vi "is_bool.vi"(11 "data in":string) -> (1 "confirmed?":bool, 3 "data out":variant)   [LabVIEW 2020, in "configuration-data.lvclass"]
uses:
  configuration-data.lvclass
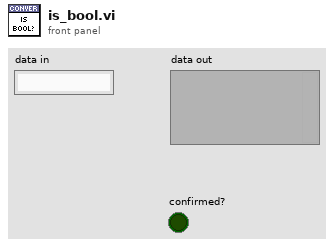
[diagram p1: front panel]
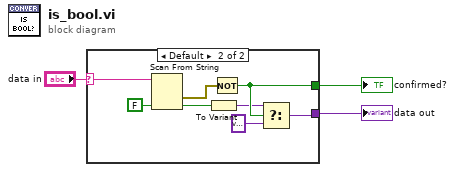
[diagram p0: block diagram]
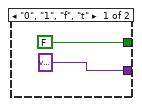
[diagram p2: hidden frame]
diagram:
  n1 = case shown="Default" "data in" {
    selector: "data in" -> [_ w13]
    tunnel: [variant w6] -> w1
    tunnel: [FALSE w10] -> w2
    frame "0", "1", "f", "t" {
    }
    frame Default {
      n2 = Scan From String(input string=w13, default 1=FALSE) -> (error out=w11:errorcluster, output 1=w9:bool)  [unwired: 3 in, 2 out]
      n3 = To Variant(anything=w9) -> (Variant=w8:variant)
      n4 = Not(x=w11) -> (.not. x?=w10:bool)
      n5 = Select(t=w8, s=w10, f=variant) -> (s? t:f=w6:variant)
    }
  }
  "confirmed?" <- w2
  "data out" <- w1
